vi "Init SequenceCountService.vi"(8 "error in (no error)":errorcluster, 11 "Vecto in":refnum<class "Vecto.lvclass">) -> (0 "error out":errorcluster, 3 "Vecto out":refnum<class "Vecto.lvclass">)   [LabVIEW 2020, in "Vecto.lvlib" / "Vecto.lvclass"]
uses:
  Vecto.lvclass
  Vecto.lvclass/Vecto.ctl
  SequenceCountService/SequenceCountService.lvclass
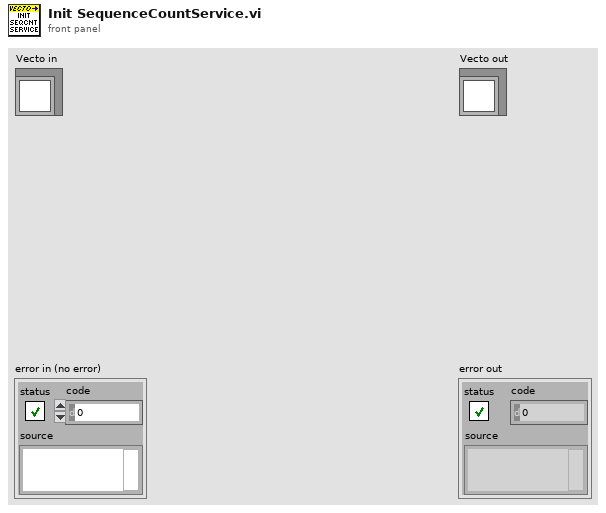
[diagram p1: front panel]
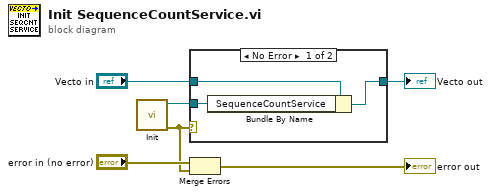
[diagram p0: block diagram]
diagram:
  n1 = call "Init.vi"() -> ("error out"=w1:errorcluster, "SequenceCountService out"=w5:refnum<class "SequenceCountService.lvclass">)  [unwired: 10 in]
  n2 = case shown="No Error" w1 {
    tunnel: "Vecto in" -> [w7 w10]
    tunnel: w5 -> [w9 _]
    tunnel: [w8 w10] -> w2
    frame No Error {
      n3 = Bundle By Name(cluster=w7, "SequenceCountService"=w9) -> (w8:refnum<class "Vecto.lvclass">)
    }
    frame Error {
    }
  }
  "Vecto out" <- w2
  n4 = Merge Errors("error in (no error)", w1) -> (→"error out":errorcluster)
